vi "COM Channel Query.vi"(0 "VISA Refnum in":refnum<visa-resource-name>, 3 "Channel":u16(ring)=1 items=["Channel 1"=1, "Channel 2"=2, "Channel 3"=3, "Channel 4"=4, "Channel 5"=5, "Channel 6"=6, "Channel 7"=7, "Channel 8"=8], 7 "error in (no error)":errorcluster) -> (20 "Channel":u16(ring)=1 items=["Channel 1"=1, "Channel 2"=2, "Channel 3"=3, "Channel 4"=4, "Channel 5"=5, "Channel 6"=6, "Channel 7"=7, "Channel 8"=8], 21 "Gain":u16(ring)=1 items=["1x"=1, "10x"=2, "100x"=3, "1000x"=4, "10000x"=5], 22 "Coupling":u16(ring)=1 items=["AC"=1, "DC"=2], 23 "Bandwidth Filter":u16(ring)=2 items=["OFF"=1, "ON"=2], 24 "Input Coupling":u16(ring)=3 items=["Off (both off)"=1, "SE + (- grounded)"=2, "SE - (+ grounded)"=3, "Diff (both on)"=4], 25 "Shunt Resistor":u16(ring)=1 items=["Open"=1, "50 Ohms"=2, "500 Ohms"=3, "5k Ohms"=4, "50k Ohms"=5], 27 "error out":errorcluster)   [LabVIEW 2013]
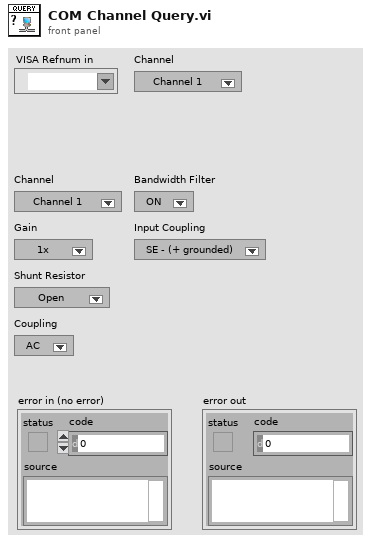
[diagram p1: front panel]
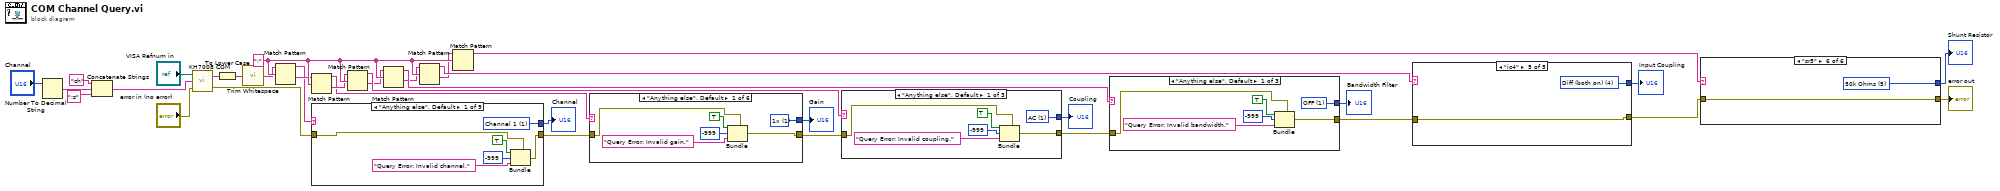
[diagram p0: block diagram]
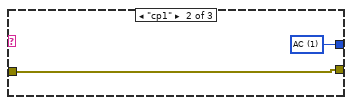
[diagram p2: hidden frame]
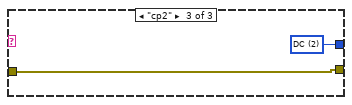
[diagram p3: hidden frame]
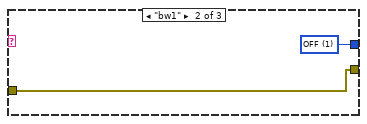
[diagram p4: hidden frame]
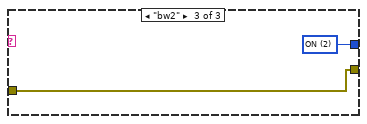
[diagram p5: hidden frame]
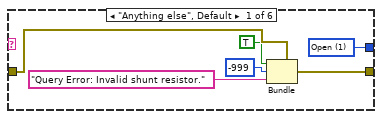
[diagram p6: hidden frame]
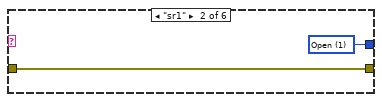
[diagram p7: hidden frame]
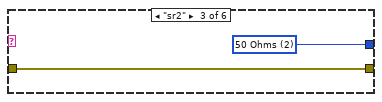
[diagram p8: hidden frame]
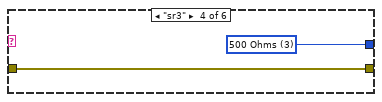
[diagram p9: hidden frame]
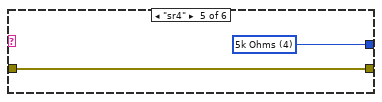
[diagram p10: hidden frame]
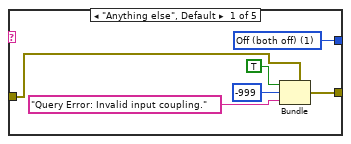
[diagram p11: hidden frame]
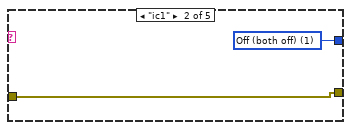
[diagram p12: hidden frame]
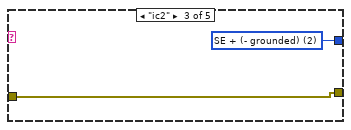
[diagram p13: hidden frame]
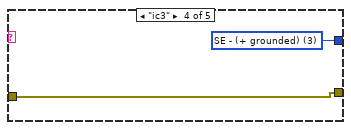
[diagram p14: hidden frame]
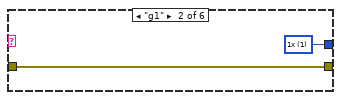
[diagram p15: hidden frame]
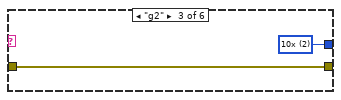
[diagram p16: hidden frame]
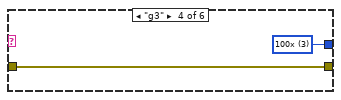
[diagram p17: hidden frame]
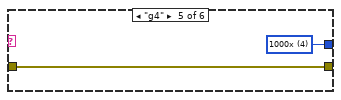
[diagram p18: hidden frame]
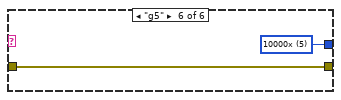
[diagram p19: hidden frame]
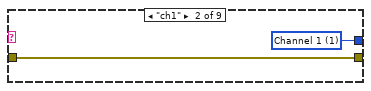
[diagram p20: hidden frame]
diagram:
  w20 = ";" ("search string/char (-)")
  n1 = Number To Decimal String(number="Channel") -> (decimal integer string=w31:string)  [unwired: 1 in]
  n2 = Concatenate Strings("ch" ("string"), w31, ";s" ("string")) -> (w33:string)
  n3 = call <vilib>:"KH7008 COM.vi"("error in (no error)"="error in (no error)", "Command"=w33, "VISA Refnum in"="VISA Refnum in") -> ("error out"=w35:errorcluster, "Response"=w12:string)
  n4 = To Lower Case(string=w12) -> (all lower case string=w10:string)
  n5 = call <vilib>:"Trim Whitespace.vi"("string"=w10) -> ("trimmed string"=w11:string)  [unwired: 1 in]
  n6 = Match Pattern(string=w11, regular expression=w20) -> (before substring=w9:string, after substring=w14:string)  [unwired: 1 in, 2 out]
  n7 = Match Pattern(string=w14, regular expression=w20) -> (before substring=w15:string, after substring=w16:string)  [unwired: 1 in, 2 out]
  n8 = case shown="\"Anything else\", Default" w9 {
    tunnel: [w41 w43 w45 w46 w49 w51 w53 w55 w57] -> w2
    tunnel: w35 -> [w40 w42 w44 w47 w48 w50 w52 w54 w56]
    tunnel: [w36 w42 w44 w47 w48 w50 w52 w54 w56] -> w13
    frame "Anything else", Default {
      w41 = u16 1 items=["Channel 1"=1, "Channel 2"=2, "Channel 3"=3, "Channel 4"=4, "Channel 5"=5, "Channel 6"=6, "Channel 7"=7, "Channel 8"=8] ("Channel")
      n9 = Bundle(cluster=w40, "status"=TRUE, "code"=-999, "source"="Query Error: Invalid channel.") -> (w36:errorcluster)
    }
    frame "ch1" {
      w43 = u16 1 items=["Channel 1"=1, "Channel 2"=2, "Channel 3"=3, "Channel 4"=4, "Channel 5"=5, "Channel 6"=6, "Channel 7"=7, "Channel 8"=8] ("Channel")
    }
    frame "ch2" {
      w45 = u16 2 items=["Channel 1"=1, "Channel 2"=2, "Channel 3"=3, "Channel 4"=4, "Channel 5"=5, "Channel 6"=6, "Channel 7"=7, "Channel 8"=8] ("Channel")
    }
    frame "ch3" {
      w46 = u16 3 items=["Channel 1"=1, "Channel 2"=2, "Channel 3"=3, "Channel 4"=4, "Channel 5"=5, "Channel 6"=6, "Channel 7"=7, "Channel 8"=8] ("Channel")
    }
    frame "ch4" {
      w49 = u16 4 items=["Channel 1"=1, "Channel 2"=2, "Channel 3"=3, "Channel 4"=4, "Channel 5"=5, "Channel 6"=6, "Channel 7"=7, "Channel 8"=8] ("Channel")
    }
    frame "ch5" {
      w51 = u16 5 items=["Channel 1"=1, "Channel 2"=2, "Channel 3"=3, "Channel 4"=4, "Channel 5"=5, "Channel 6"=6, "Channel 7"=7, "Channel 8"=8] ("Channel")
    }
    frame "ch6" {
      w53 = u16 6 items=["Channel 1"=1, "Channel 2"=2, "Channel 3"=3, "Channel 4"=4, "Channel 5"=5, "Channel 6"=6, "Channel 7"=7, "Channel 8"=8] ("Channel")
    }
    frame "ch7" {
      w55 = u16 7 items=["Channel 1"=1, "Channel 2"=2, "Channel 3"=3, "Channel 4"=4, "Channel 5"=5, "Channel 6"=6, "Channel 7"=7, "Channel 8"=8] ("Channel")
    }
    frame "ch8" {
      w57 = u16 8 items=["Channel 1"=1, "Channel 2"=2, "Channel 3"=3, "Channel 4"=4, "Channel 5"=5, "Channel 6"=6, "Channel 7"=7, "Channel 8"=8] ("Channel")
    }
  }
  "Channel" <- w2
  n10 = Match Pattern(string=w16, regular expression=w20) -> (before substring=w24:string, after substring=w17:string)  [unwired: 1 in, 2 out]
  n11 = Match Pattern(string=w17, regular expression=w20) -> (before substring=w25:string, after substring=w18:string)  [unwired: 1 in, 2 out]
  n12 = Match Pattern(string=w18, regular expression=w20) -> (before substring=w27:string, after substring=w19:string)  [unwired: 1 in, 2 out]
  n13 = Match Pattern(string=w19, regular expression=w20) -> (before substring=w21:string)  [unwired: 1 in, 3 out]
  n14 = case shown="\"Anything else\", Default" w15 {
    tunnel: [w58 w64 w66 w68 w70 w72] -> w3
    tunnel: w13 -> [w63 w65 w67 w69 w71 w73]
    tunnel: [w59 w65 w67 w69 w71 w73] -> w22
    frame "Anything else", Default {
      w58 = u16 1 items=["1x"=1, "10x"=2, "100x"=3, "1000x"=4, "10000x"=5] ("Gain")
      n15 = Bundle(cluster=w63, "status"=TRUE, "code"=-999, "source"="Query Error: Invalid gain.") -> (w59:errorcluster)
    }
    frame "g1" {
      w64 = u16 1 items=["1x"=1, "10x"=2, "100x"=3, "1000x"=4, "10000x"=5] ("Gain")
    }
    frame "g2" {
      w66 = u16 2 items=["1x"=1, "10x"=2, "100x"=3, "1000x"=4, "10000x"=5] ("Gain")
    }
    frame "g3" {
      w68 = u16 3 items=["1x"=1, "10x"=2, "100x"=3, "1000x"=4, "10000x"=5] ("Gain")
    }
    frame "g4" {
      w70 = u16 4 items=["1x"=1, "10x"=2, "100x"=3, "1000x"=4, "10000x"=5] ("Gain")
    }
    frame "g5" {
      w72 = u16 5 items=["1x"=1, "10x"=2, "100x"=3, "1000x"=4, "10000x"=5] ("Gain")
    }
  }
  "Gain" <- w3
  n16 = case shown="\"Anything else\", Default" w24 {
    tunnel: [w74 w80 w82] -> w4
    tunnel: w22 -> [w79 w81 w83]
    tunnel: [w75 w81 w83] -> w23
    frame "Anything else", Default {
      w74 = u16 1 items=["AC"=1, "DC"=2] ("Coupling")
      n17 = Bundle(cluster=w79, "status"=TRUE, "code"=-999, "source"="Query Error: Invalid coupling.") -> (w75:errorcluster)
    }
    frame "cp1" {
      w80 = u16 1 items=["AC"=1, "DC"=2] ("Coupling")
    }
    frame "cp2" {
      w82 = u16 2 items=["AC"=1, "DC"=2] ("Coupling")
    }
  }
  "Coupling" <- w4
  n18 = case shown="\"Anything else\", Default" w25 {
    tunnel: [w84 w90 w92] -> w5
    tunnel: w23 -> [w89 w91 w93]
    tunnel: [w85 w91 w93] -> w26
    frame "Anything else", Default {
      w84 = u16 1 items=["OFF"=1, "ON"=2] ("Bandwidth Filter")
      n19 = Bundle(cluster=w89, "status"=TRUE, "code"=-999, "source"="Query Error: Invalid bandwidth.") -> (w85:errorcluster)
    }
    frame "bw1" {
      w90 = u16 1 items=["OFF"=1, "ON"=2] ("Bandwidth Filter")
    }
    frame "bw2" {
      w92 = u16 2 items=["OFF"=1, "ON"=2] ("Bandwidth Filter")
    }
  }
  "Bandwidth Filter" <- w5
  n20 = case shown="\"ic4\"" w27 {
    tunnel: [w94 w100 w102 w104 w106] -> w6
    tunnel: w26 -> [w99 w101 w103 w105 w107]
    tunnel: [w95 w101 w103 w105 w107] -> w28
    frame "Anything else", Default {
      w94 = u16 1 items=["Off (both off)"=1, "SE + (- grounded)"=2, "SE - (+ grounded)"=3, "Diff (both on)"=4] ("Input Coupling")
      n21 = Bundle(cluster=w99, "status"=TRUE, "code"=-999, "source"="Query Error: Invalid input coupling.") -> (w95:errorcluster)
    }
    frame "ic1" {
      w100 = u16 1 items=["Off (both off)"=1, "SE + (- grounded)"=2, "SE - (+ grounded)"=3, "Diff (both on)"=4] ("Input Coupling")
    }
    frame "ic2" {
      w102 = u16 2 items=["Off (both off)"=1, "SE + (- grounded)"=2, "SE - (+ grounded)"=3, "Diff (both on)"=4] ("Input Coupling")
    }
    frame "ic3" {
      w104 = u16 3 items=["Off (both off)"=1, "SE + (- grounded)"=2, "SE - (+ grounded)"=3, "Diff (both on)"=4] ("Input Coupling")
    }
    frame "ic4" {
      w106 = u16 4 items=["Off (both off)"=1, "SE + (- grounded)"=2, "SE - (+ grounded)"=3, "Diff (both on)"=4] ("Input Coupling")
    }
  }
  "Input Coupling" <- w6
  n22 = case shown="\"sr5\"" w21 {
    tunnel: [w108 w114 w116 w118 w120 w122] -> w7
    tunnel: w28 -> [w113 w115 w117 w119 w121 w123]
    tunnel: [w109 w115 w117 w119 w121 w123] -> w29
    frame "Anything else", Default {
      w108 = u16 1 items=["Open"=1, "50 Ohms"=2, "500 Ohms"=3, "5k Ohms"=4, "50k Ohms"=5] ("Shunt Resistor")
      n23 = Bundle(cluster=w113, "status"=TRUE, "code"=-999, "source"="Query Error: Invalid shunt resistor.") -> (w109:errorcluster)
    }
    frame "sr1" {
      w114 = u16 1 items=["Open"=1, "50 Ohms"=2, "500 Ohms"=3, "5k Ohms"=4, "50k Ohms"=5] ("Shunt Resistor")
    }
    frame "sr2" {
      w116 = u16 2 items=["Open"=1, "50 Ohms"=2, "500 Ohms"=3, "5k Ohms"=4, "50k Ohms"=5] ("Shunt Resistor")
    }
    frame "sr3" {
      w118 = u16 3 items=["Open"=1, "50 Ohms"=2, "500 Ohms"=3, "5k Ohms"=4, "50k Ohms"=5] ("Shunt Resistor")
    }
    frame "sr4" {
      w120 = u16 4 items=["Open"=1, "50 Ohms"=2, "500 Ohms"=3, "5k Ohms"=4, "50k Ohms"=5] ("Shunt Resistor")
    }
    frame "sr5" {
      w122 = u16 5 items=["Open"=1, "50 Ohms"=2, "500 Ohms"=3, "5k Ohms"=4, "50k Ohms"=5] ("Shunt Resistor")
    }
  }
  "error out" <- w29
  "Shunt Resistor" <- w7
